vi "Initialize.vi"(8 "error in (no error)":errorcluster, 11 "CCD in":refnum<class "Motor.lvclass">) -> (0 "error out":errorcluster, 3 "CCD out":refnum<class "Motor.lvclass">)   [LabVIEW 2016, in "Hardware.lvlib" / "Motor.lvlib" / "Motor.lvclass"]
uses:
  <userlib>/Common Components/Hardware/Motor/Motor/Motor.lvclass
  C:/Program Files (x86)/National Instruments/LabVIEW 2016/user.lib/Common Components/Hardware/Abstract Hardware/Hardware.lvclass
  <userlib>/Common Components/Hardware/Abstract Hardware/Hardware.lvclass/Hardware.ctl
  <userlib>/Common Components/Hardware/Motor/Motor/Motor.lvclass/Motor.ctl
  <userlib>/Common Components/Hardware/Abstract Hardware/Read Label.vi
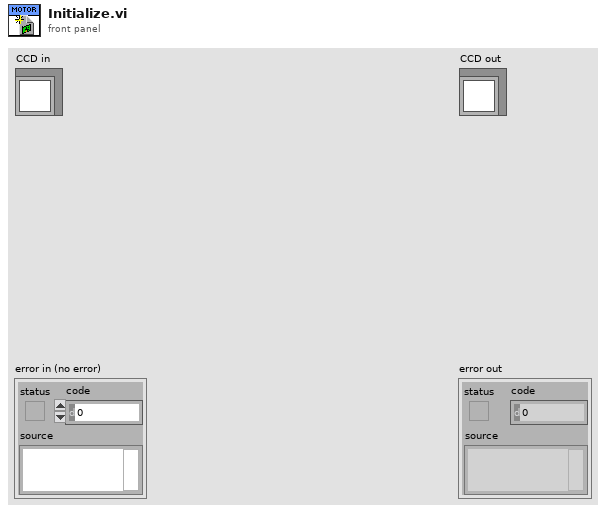
[diagram p1: front panel]
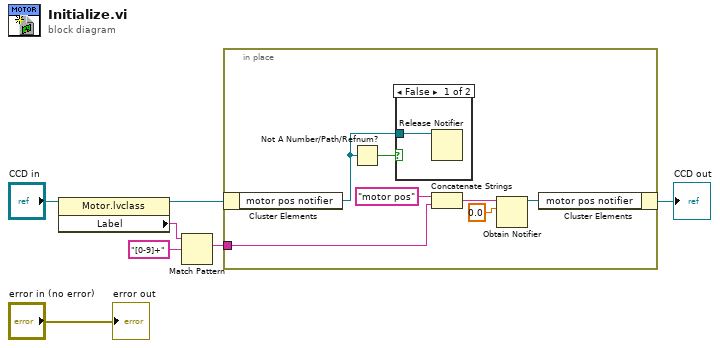
[diagram p0: block diagram]
diagram:
  n1 = property class="Motor.lvclass"(reference="CCD in") -> (reference out=w4:refnum<class "Motor.lvclass">, "Label"=w3:string)  [unwired: 1 in, 1 out]
  n2 = Match Pattern(string=w3, regular expression="[0-9]+") -> (match substring=w2:string)  [unwired: 1 in, 3 out]
  n3 = in-place {
    in-place-border: w2 -> [w8]
    n4 = in-place-cluster #1(w4) -> ("motor pos notifier"=w10:refnum<notifier>)
    n5 = Not A Number/Path/Refnum?(number/path/refnum=w10) -> (NaN/Path/Refnum?=w11:bool)
    n6 = case shown="False" w11 {
      tunnel: w10 -> [w15 _]
      frame False {
        n7 = Release Notifier(notifier=w15) -> ()  [unwired: 2 in, 3 out]
      }
      frame True {
      }
    }
    n8 = Concatenate Strings("motor pos" ("name (unnamed)"), w8) -> (w9:string)
    n9 = Obtain Notifier(name (unnamed)=w9, notification data type=0.0 ("pos in motor (pulses)")) -> (notifier out=w12:refnum<notifier>)  [unwired: 2 in, 2 out]
    n10 = in-place-cluster #1("motor pos notifier"=w12) -> (→"CCD out":refnum<class "Motor.lvclass">)
  }
  "error out" <- "error in (no error)"
